vi "Function_PatternMach.vi"(8 "Error in":errorcluster, 9 "Data Cluster In":cluster{"Name":string, "Variant In":variant}, 10 "Template Image":T3, 11 "Image Src In":T3) -> (0 "Error out":errorcluster, 1 "CoordSys Out":T1 {"Measurement System"."Axis Reference" items=["Direct", "Indirect"]; "Measurement System"."Angle (deg)" format="%.2f"; "Measurement System"."Origin"."Y" format="%.2f"; "Measurement System"."Origin"."X" format="%.2f"; "Reference System"."Axis Reference" items=["Direct", "Indirect"]; "Reference System"."Angle (deg)" format="%.2f"; "Reference System"."Origin"."Y" format="%.2f"; "Reference System"."Origin"."X" format="%.2f"}, 2 "Data Cluster Out":cluster{"Name":string, "Variant In":variant}, 3 "Matches":T2(array[cluster]) {"Bounding Box"."y" format="%.2f"; "Bounding Box"."x" format="%.2f"; "Position"."y" format="%.2f"; "Position"."x" format="%.2f"; "Score" format="%.2f"; "Scale" format="%.2f"; "Angle" format="%.2f"}, 4 "Result(PM)":cluster{"Name":string, "NG?":bool, "Score":dbl})   [LabVIEW 2013]
uses:
  <vilib>/vision/Image Controls.llb/IMAQ Image.ctl
  Control/Control Pattern Match.ctl
  <vilib>/vision/NI_Vision_Development_Module.lvlib
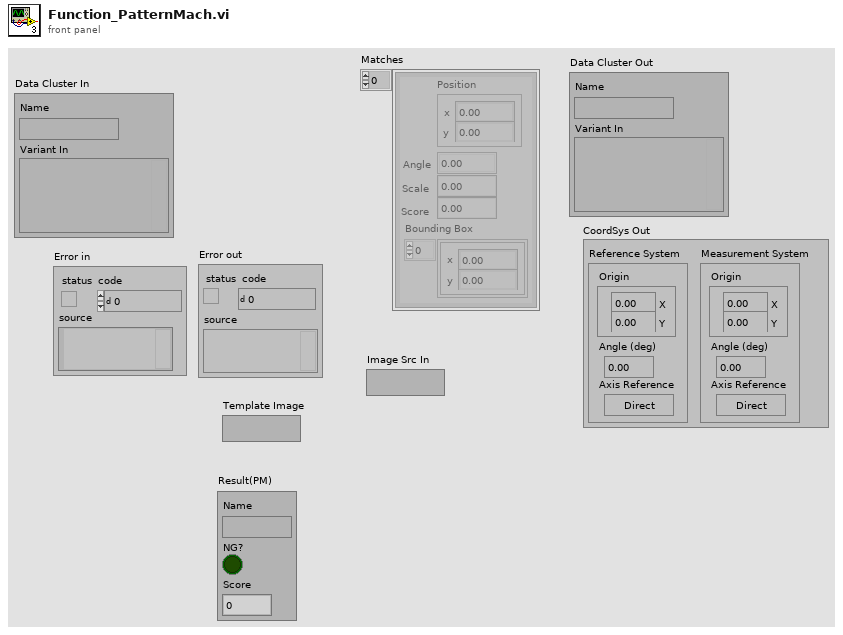
[diagram p1: front panel]
types:
  T1 = typedef "IMAQ Coordinate System" = cluster{"Reference System":cluster{"Origin":cluster{"X":sgl, "Y":sgl}, "Angle (deg)":sgl, "Axis Reference":u32}, "Measurement System":cluster{"Origin":cluster{"X":sgl, "Y":sgl}, "Angle (deg)":sgl, "Axis Reference":u32}}
  T2 = cluster{"Position":cluster{"x":sgl, "y":sgl}, "Angle":sgl, "Scale":sgl, "Score":sgl, "Bounding Box":cluster{"x":sgl, "y":sgl}[]}[]
  T3 = typedef "IMAQ Image.ctl" = refnum<image>
  T4 = typedef "Control Pattern Match.ctl" = cluster{"ROI_尋樣本":T5, "Algorithm":i32, "Parameters":cluster{"Number of Matches Requested":i32, "Minimum Match Score":sgl, "Angle Ranges":cluster{"Start Angle":sgl, "End Angle":sgl}[]}, "Mode":u16, "CoordSys In":T1}
  T5 = typedef "ROI Descriptor" = cluster{"Global Rectangle":i32[], "Contours":cluster{"ID":enum32{"External", "Internal"}, "Type":u32, "Coordinates":i32[]}[]}
  T6 = cluster{"Number of Matches Requested":i32, "Minimum Match Score":sgl, "Angle Ranges":cluster{"Start Angle":sgl, "End Angle":sgl}[]}
  T7 = cluster{"Position":cluster{"x":sgl, "y":sgl}, "Angle":sgl, "Scale":sgl, "Score":sgl, "Bounding Box":cluster{"x":sgl, "y":sgl}[]}
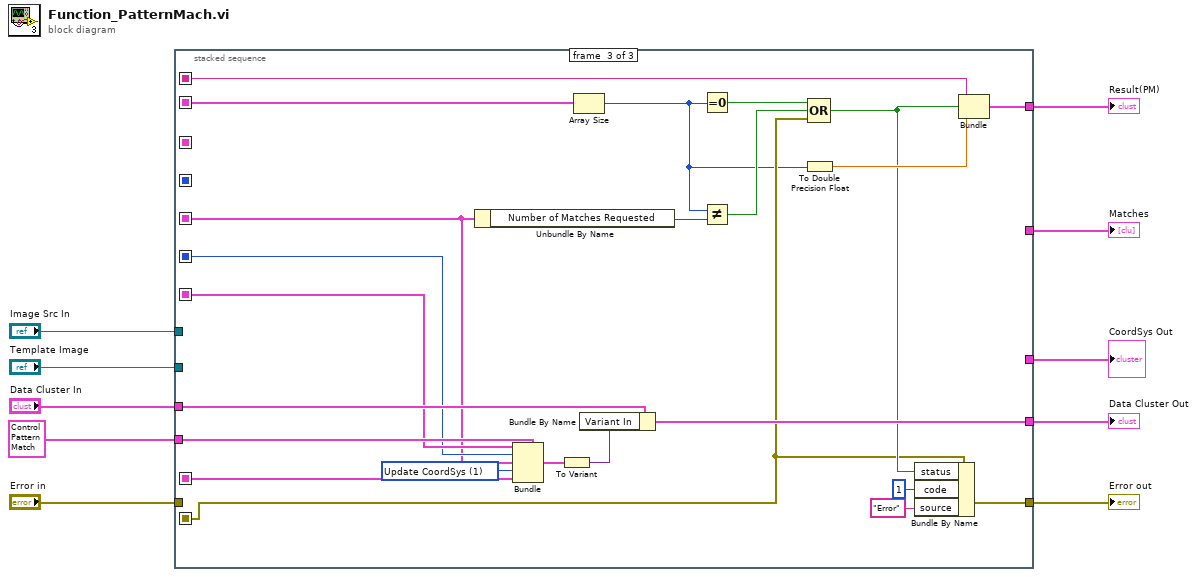
[diagram p0: block diagram]
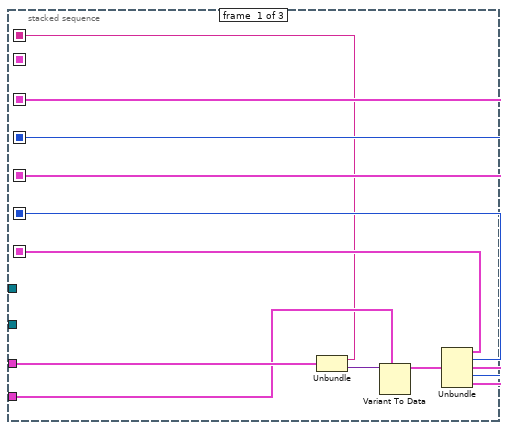
[diagram p2: hidden frame]
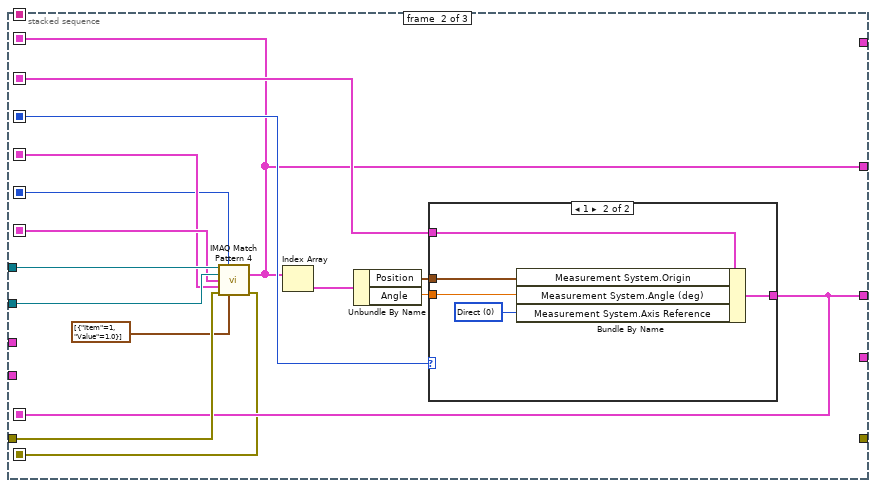
[diagram p3: hidden frame]
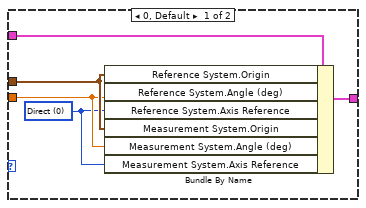
[diagram p4: hidden frame]
diagram:
  n1 = stacked-sequence {
    seq-local: [w18 _ _] -> [_ w29 w65]
    seq-local: [w17 _ _] -> [_ w25 w64]
    seq-local: [w15 _ _] -> [_ w28 w50]
    seq-local: [w16 _ _] -> [_ w27 _]
    seq-local: [w14 _ _] -> [_ w26 _]
    seq-local: [_ w24 _] -> [_ _ w66]
    seq-local: [_ w21 _] -> [_ _ w61]
    seq-local: [_ w22 _] -> [_ _ w47]
    seq-local: [w11 _ _] -> [_ _ w59]
    tunnel: "Error in" -> [_ w32 _]
    tunnel: [_ _ w56] -> w10
    tunnel: "Template Image" -> [_ w31 _]
    tunnel: "Image Src In" -> [_ w30 _]
    tunnel: [_ w21 _] -> w7
    tunnel: "Data Cluster In" -> [w13 _ w67]
    tunnel: T4 {"ROI_尋樣本"={"Global Rectangle"=[], "Contours"=[]}, "Algorithm"=0, "Parameters"={"Number of Matches Requested"=1, "Minimum Match Score"=800.0, "Angle Ranges"=[]}, "Mode"=0, "CoordSys In"={"Reference System"={"Origin"={"X"=0.0, "Y"=0.0}, "Angle (deg)"=0.0, "Axis Reference"=0}, "Measurement System"={"Origin"={"X"=0.0, "Y"=0.0}, "Angle (deg)"=0.0, "Axis Reference"=0}}} ("模型_Setting") -> [w12 _ w68]
    tunnel: [_ _ w63] -> w4
    tunnel: [_ w24 _] -> w3
    tunnel: [_ _ w60] -> w2
    frame #0 {
      n2 = Unbundle(w13) -> ("Name"=w11:string, "Variant In"=w20:variant)
      n3 = Variant To Data(type=w12, Variant=w20) -> (data=w19:T4)  [unwired: 1 in, 1 out]
      n4 = Unbundle(w19) -> ("ROI_尋樣本"=w18:T5, "Algorithm"=w17:i32, "Parameters"=w15:T6, "Mode"=w16:u16, "CoordSys In"=w14:T1)
    }
    frame #1 {
      n5 = call "IMAQ Match Pattern 4"("Image"=w30, "Algorithm"=w25, "Template Image"=w31, "ROI Descriptor"=w29, "Parameters"=w28, "error in (no error)"=w32, "Advanced Options"=cluster{"Item":u16, "Value":dbl}[] [{"Item"=1, "Value"=1.0}]) -> ("Matches (pixel)"=w21:T2, "error out"=w22:errorcluster)  [unwired: 4 in, 3 out]
      n6 = Index Array(array=w21) -> (element=w35:T7)  [unwired: 1 in]
      n7 = Unbundle By Name(w35) -> ("Position"=w33:cluster{"x":sgl, "y":sgl}, "Angle"=w34:sgl)
      n8 = case shown="1" w27 {
        tunnel: w33 -> [w38 w43]
        tunnel: [w40 w45] -> w24
        tunnel: w34 -> [w37 w42]
        tunnel: w26 -> [w39 w44]
        frame 0, Default {
          w36 = u32 0 items=["Direct", "Indirect"] ("Axis Reference")
          n9 = Bundle By Name(cluster=w39, "Reference System.Origin"=w38, "Reference System.Angle (deg)"=w37, "Reference System.Axis Reference"=w36, "Measurement System.Origin"=w38, "Measurement System.Angle (deg)"=w37, "Measurement System.Axis Reference"=w36) -> (w40:T1)
        }
        frame 1 {
          w41 = u32 0 items=["Direct", "Indirect"] ("Axis Reference")
          n10 = Bundle By Name(cluster=w44, "Measurement System.Origin"=w43, "Measurement System.Angle (deg)"=w42, "Measurement System.Axis Reference"=w41) -> (w45:T1)
        }
      }
    }
    frame #2 {
      w62 = u16 1 items=["Find Reference", "Update CoordSys"] ("Mode")
      n11 = Unbundle By Name(w50) -> ("Number of Matches Requested"=w49:i32)
      n12 = Bundle(cluster=w68, "ROI_尋樣本"=w65, "Algorithm"=w64, "Parameters"=w50, "Mode"=w62, "CoordSys In"=w66) -> (w52:T4)
      n13 = To Variant(anything=w52) -> (Variant=w51:variant)
      n14 = Array Size(array=w61) -> (size(s)=w46:i32)
      n15 = Bundle By Name(cluster=w67, "Variant In"=w51) -> (w63:cluster{"Name":string, "Variant In":variant})
      n16 = Equal To 0?(x=w46) -> (x = 0?=w58:bool)
      n17 = Not Equal?(x=w46, y=w49) -> (x != y?=w48:bool)
      n18 = To Double Precision Float(number=w46) -> (double precision float=w57:dbl)
      n19 = Compound Arithmetic op=OR(w58, w48, w47) -> (w55:bool)
      n20 = Bundle By Name(cluster=w47, "status"=w55, "code"=1, "source"="Error") -> (w56:errorcluster)
      n21 = Bundle("Name"=w59, w55, w57) -> (w60:cluster{"Name":string, bool, dbl})  [unwired: 1 in]
    }
  }
  "Error out" <- w10
  "Matches" <- w7
  "Data Cluster Out" <- w4
  "CoordSys Out" <- w3
  "Result(PM)" <- w2
